vi "WFS Revision Query.vi"(8 "error in (no error)":errorcluster {"code" format="%.0x"}, 11 "instrument handle":refnum<visa-resource-name>) -> (0 "error out":errorcluster {"code" format="%.0x"}, 1 "Firmware Revision":string, 2 "Instrument Driver Revision":string, 3 "instrument handle out":refnum<visa-resource-name>)   [LabVIEW 2020]
doc: "This VI returns the revision of the instrument driver and the firmware revision of the instrument being used."
uses:
  WFS_32.dll
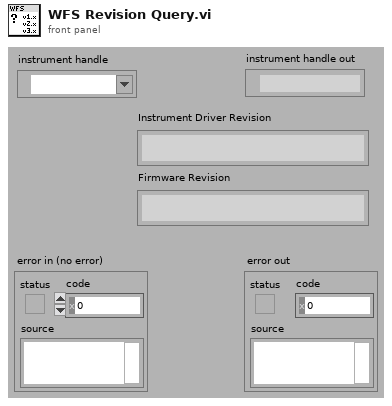
[diagram p1: front panel]
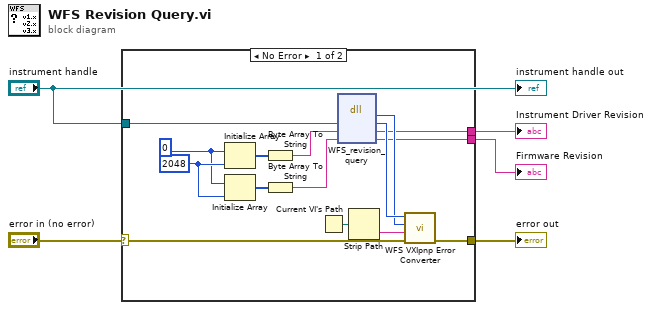
[diagram p0: block diagram]
diagram:
  n1 = case shown="No Error" "error in (no error)" {
    selector: "error in (no error)" -> [w9 w21]
    tunnel: [w8 w21] -> w4
    tunnel: "instrument handle" -> [w13 _]
    tunnel: [w7 _] -> w2
    tunnel: [w6 _] -> w1
    frame No Error {
      w14 = u8 0
      w15 = 2048 ("size of firmware revision")
      n2 = Initialize Array(w14, w15) -> (w20:u8[])
      n3 = Initialize Array(w14, w15) -> (w19:u8[])
      n4 = Byte Array To String(unsigned byte array=w20) -> (string=w18:string)
      n5 = Byte Array To String(unsigned byte array=w19) -> (string=w17:string)
      n6 = Current VI's Path() -> (path=w16:path)
      n7 = dll-call lib="WFS_*.*" fn="WFS_revision_query"("instrument handle"=w13, "instrument driver revision"=w18, "firmware revision"=w17) -> ("Status"=w11:i32, "instrument handle"=w12:u32, "instrument driver revision"=w7:string, "firmware revision"=w6:string)  [unwired: 3 in, 2 out]
      n8 = Strip Path(path=w16) -> (name=w10:string)  [unwired: 1 out]
      n9 = call "WFS VXIpnp Error Converter.vi"("error in (no error)"=w9, "Name Of VI (\"\")"=w10, "CVI Error Code (0)"=w11, "instrument handle"=w12) -> ("error out"=w8:errorcluster)  [unwired: 6 in, 1 out]
    }
    frame Error {
    }
  }
  "error out" <- w4
  "Instrument Driver Revision" <- w2
  "Firmware Revision" <- w1
  "instrument handle out" <- "instrument handle"
